vi "Read Conversion Time.vi"(8 "error in":errorcluster, 11 "9224 in":refnum<class "9224.lvclass">) -> (0 "error out":errorcluster, 2 "Conversion Time":T1 items=["High Speed (1k S/s)", "Medium Speed (100 S/s)", "Medium Resolution (50/60Hz Rejection - 12 S/s)", "High Resolution (50/60Hz rejection - 2 S/s)"], 3 "9224 out":refnum<class "9224.lvclass">)   [LabVIEW 2019, in "Modules.lvlib" / "9224.lvclass"]
uses:
  9224.lvclass
  Conversion Time.ctl
  9224.lvclass/9224.ctl
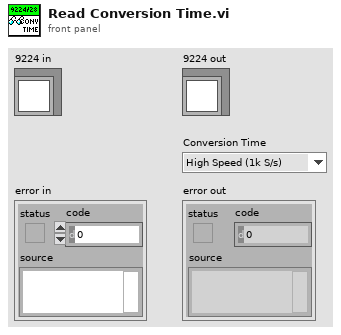
[diagram p1: front panel]
types:
  T1 = typedef "Modules.lvlib/9224.lvclass/Conversion Time.ctl" = u16
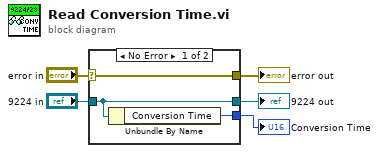
[diagram p0: block diagram]
diagram:
  n1 = case shown="No Error" "error in" {
    selector: "error in" -> [w8 w9]
    tunnel: [w8 w9] -> w4
    tunnel: [w7 w10] -> w2
    tunnel: "9224 in" -> [w7 w10]
    tunnel: [w6 _] -> w1
    frame No Error {
      n2 = Unbundle By Name(w7) -> ("Conversion Time"=w6:T1)
    }
    frame Error {
    }
  }
  "error out" <- w4
  "9224 out" <- w2
  "Conversion Time" <- w1
